vi "SetRoi.vi"() -> ()   [LabVIEW 2013]
panel:
  in  "SetRoi":bool
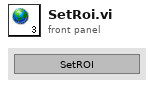
[diagram p1: front panel]
diagram:
